vi "Chronos TDMS Sort Groups and Channels.vi"(8 "error in (no error)":errorcluster, 11 "Channels":T1[](array[typedef])) -> (0 "error out":errorcluster, 2 "TDMS Ch List":cluster{string[]}[](array[cluster]), 3 "TDMS Groups":string[](array[string]))   [LabVIEW 2021]
uses:
  typedefs/Chronos cluster Channel.ctl
  typedefs/Chronos cluster Hardware Configuration Physical.ctl
  Subsystem Modules/Chronos enum Device Hardware Type.ctl
  typedefs/Chronos cluster Scaling.ctl
  typedefs/Chronos enum Scaling Type.ctl
  typedefs/Chronos cluster Limits.ctl
  typedefs/Chronos cluster Alarm.ctl
  typedefs/Chronos enum Alarm Action.ctl
  typedefs/Chronos cluster Channel Configuration variant.ctl
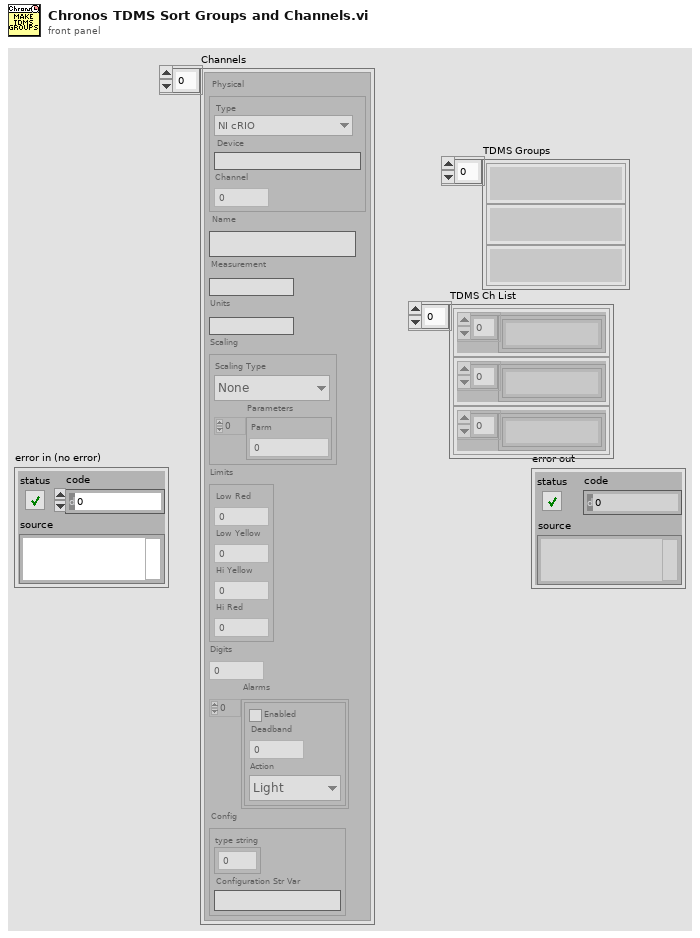
[diagram p1: front panel]
types:
  T1 = typedef "Chronos cluster Channel.ctl" = cluster{"Physical":T2, "Name":string, "Measurement":string, "Units":string, "Scaling":T4, "Limits":T6, "Digits":i32, "Alarms":T7[], "Config":T9}
  T2 = typedef "Chronos cluster Hardware Configuration Physical.ctl" = cluster{"Type":T3, "Device":string, "Channel":i32}
  T3 = typedef "Chronos enum Device Hardware Type.ctl" = enum16{"NI cRIO", "Keithley 3706"}
  T4 = typedef "Chronos cluster Scaling.ctl" = cluster{"Scaling Type":T5, "Parameters":dbl[]}
  T5 = typedef "Chronos enum Scaling Type.ctl" = enum16{"None", "Polynomial"}
  T6 = typedef "Chronos cluster Limits.ctl" = cluster{"Low Red":dbl, "Low Yellow":dbl, "Hi Yellow":dbl, "Hi Red":dbl}
  T7 = typedef "Chronos cluster Alarm.ctl" = cluster{"Enabled":bool, "Deadband":i32, "Action":T8}
  T8 = typedef "Chronos enum Alarm Action.ctl" = enum16{"Light", "Message", "Safe"}
  T9 = typedef "Chronos cluster Channel Configuration variant.ctl" = cluster{"type string":i16[], "Configuration Str Var":string}
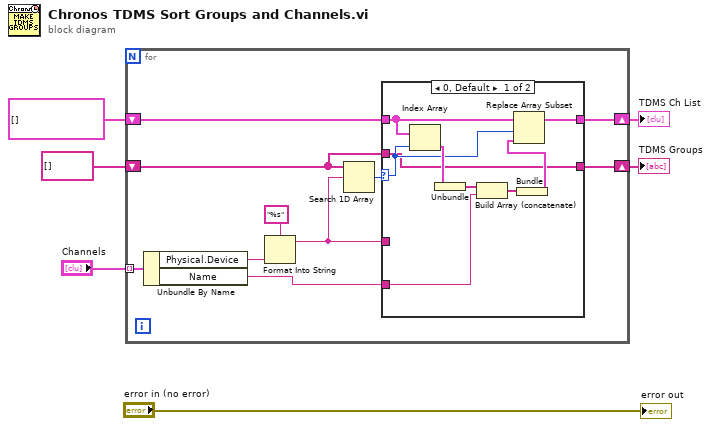
[diagram p0: block diagram]
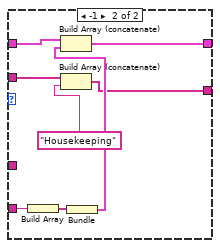
[diagram p2: hidden frame]
diagram:
  n1 = for {
    tunnel: "Channels" -> [w15] mode=indexing
    shift-right: [w7] -> w3
    shift-left: string[] [] -> [w10]
    shift-right: [w9] -> w4
    shift-left: cluster{string[]}[] [] -> [w8]
    n2 = Unbundle By Name(w15) -> ("Physical.Device"=w14:string, "Name"=w11:string)
    n3 = Format Into String(format string="%s", w14) -> (resulting string=w12:string)  [unwired: 2 in, 1 out]
    n4 = Search 1D Array(1D array=w10, element=w12) -> (index of element=w13:i32)  [unwired: 1 in]
    n5 = case shown="0, Default" w13 {
      selector: w13 -> [w19 _]
      tunnel: w12 -> [_ _]
      tunnel: w11 -> [w24 w33]
      tunnel: w10 -> [w17 w31]
      tunnel: [w18 w29] -> w9
      tunnel: w8 -> [w22 w28]
      tunnel: [w17 w27] -> w7
      frame 0, Default {
        n6 = Index Array(array=w22, index=w19) -> (element=w25:cluster{string[]})
        n7 = Unbundle(w25) -> (w23:string[])
        n8 = Build Array (concatenate)(w23, w24) -> (w21:string[])
        n9 = Bundle(w21) -> (w20:cluster{string[]})  [unwired: 1 in]
        n10 = Replace Array Subset(array=w22, new element=w20, index=w19) -> (w18:cluster{string[]}[])
      }
      frame -1 {
        n11 = Build Array(w33) -> (w32:string[])
        n12 = Build Array (concatenate)(w31, "Housekeeping") -> (w27:string[])
        n13 = Bundle(w32) -> (w30:cluster{string[]})  [unwired: 1 in]
        n14 = Build Array (concatenate)(w28, w30) -> (w29:cluster{string[]}[])
      }
    }
  }
  "TDMS Ch List" <- w4
  "TDMS Groups" <- w3
  "error out" <- "error in (no error)"
